vi "Telemetria+Datalogger.vi"() -> ()   [LabVIEW 2018]
uses:
  <vilib>/Utility/file.llb/Write Delimited Spreadsheet (string).vi
  <vilib>/Instr/_visa.llb/VISA Configure Serial Port (Instr).vi
  <vilib>/Utility/file.llb/Write Delimited Spreadsheet (I64).vi
  <vilib>/MakerHub/LINX/LMH-LINX.lvlib
panel:
  out "ITA":dbl
  out "AFR":dbl
  out "ECUS":dbl
  in  "stop":bool
  in  "VISA resource name":refnum<visa-resource-name>
  out "Loop Rate (Hz)":u32
  in  "Tab Control":T1(tab)
  out "BATT":dbl(knob) scale=0.0..14.0
  out "RPM":dbl(knob) scale=0.0..10000.0
  out "VSS1":dbl(knob) scale=0.0..200.0
  out "BATC":dbl(knob) scale=0.0..10.0
  out "VO2":dbl(knob) scale=0.0..10.0
  out "FP1":dbl(knob) scale=0.0..10.0
  out "BARO":dbl(knob) scale=0.0..100.0
  out "MAP":dbl(knob) scale=0.0..10.0
  out "CLT":dbl(slide) scale=0.0..10.0
  out "MAT":dbl(slide) scale=0.0..10.0
  out "AFC":dbl(slide) scale=0.0..10.0
  out "ADC":dbl(slide) scale=0.0..100.0
  out "WC":dbl(slide) scale=0.0..100.0
  out "VE1":dbl(slide) scale=0.0..10.0
  out "VE2":dbl(slide) scale=0.0..10.0
  out "LOAD":dbl(slide) scale=0.0..100.0
  out "KNOCK":i32(graph)
  out "TPS":i32(graph)
  out "KNOCK":string
  out "BARO":string
  in  "offset BARO":i32
  out "MAP":string
  out "RPM":string
  in  "length RPM":i32
  in  "offset RPM":i32
  out "CLT":string
  out "TPS":string
  in  "length TPS":i32
  in  "offset TPS":i32
  out "BATT":string
  in  "length BATT":i32
  in  "offset BATT":i32
  in  "length KNOCK":i32
  in  "offset KNOCK":i32
  out "MAT":string
  in  "length MAT":i32
  in  "offset MAT":i32
  out "VSS1":string
  in  "length VSS1":i32
  in  "offset VSS1":i32
  in  "length MAP":i32
  in  "offset MAP":i32
  in  "length CLT":i32
  in  "offset  CLT":i32
  in  "length BARO":i32
  out "GEAR":string
  in  "length GEAR":i32
  in  "offset GEAR":i32
  out "ENGINE":string
  in  "length ENGINE":i32
  in  "offset ENGINE":i32
  out "read buffer":string
  out "FP1":string
  in  "length FP1":i32
  in  "offset FP1":i32
  out "ECUS":string
  in  "offset ECUS":i32
  in  "length ECUS":i32
  out "AFC":string
  in  "length AFC":i32
  in  "offset AFC":i32
  out "BATC":string
  in  "length BATC":i32
  in  "offset BATC":i32
  out "VO2":string
  in  "length VO2":i32
  in  "offset VO2":i32
  out "ADC":string
  in  "length ADC":i32
  in  "offset ADC":i32
  out "WC":string
  in  "length WC":i32
  in  "offset WC":i32
  out "VE1":string
  in  "length VE1":i32
  in  "offset VE1":i32
  out "VE2":string
  in  "length VE2":i32
  in  "offset VE2":i32
  out "LOAD":string
  in  "length LOAD":i32
  in  "offset LOAD":i32
  out "AFR":string
  in  "length AFR":i32
  in  "offset AFR":i32
  out "ITA":string
  in  "length ITA":i32
  in  "offset ITA":i32
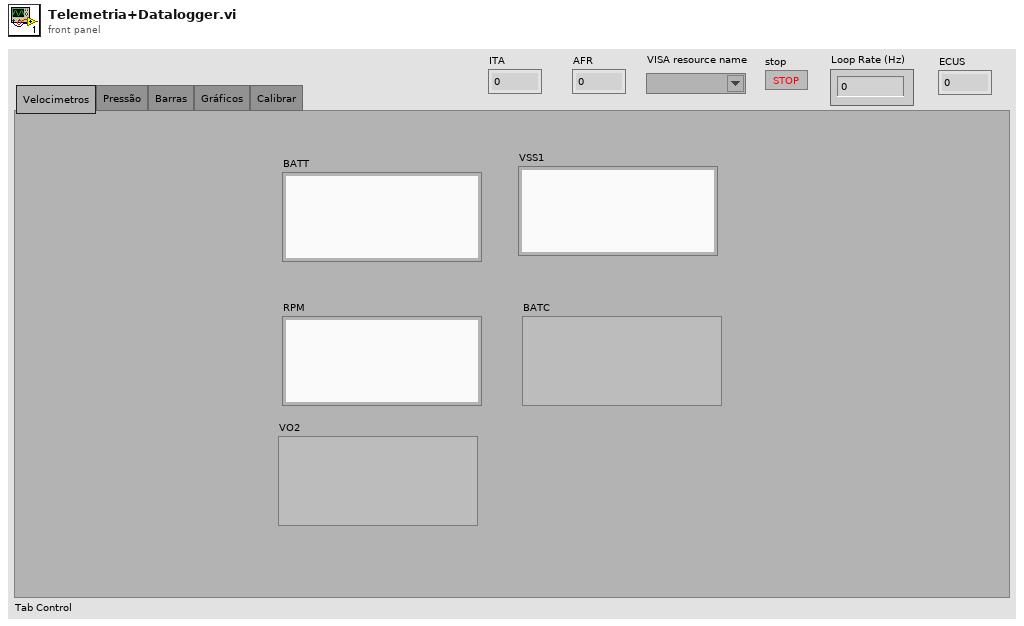
[diagram p1: front panel]
types:
  T1 = enum32{"Velocimetros", "Pressão", "Barras", "Gráficos", "Calibrar"}
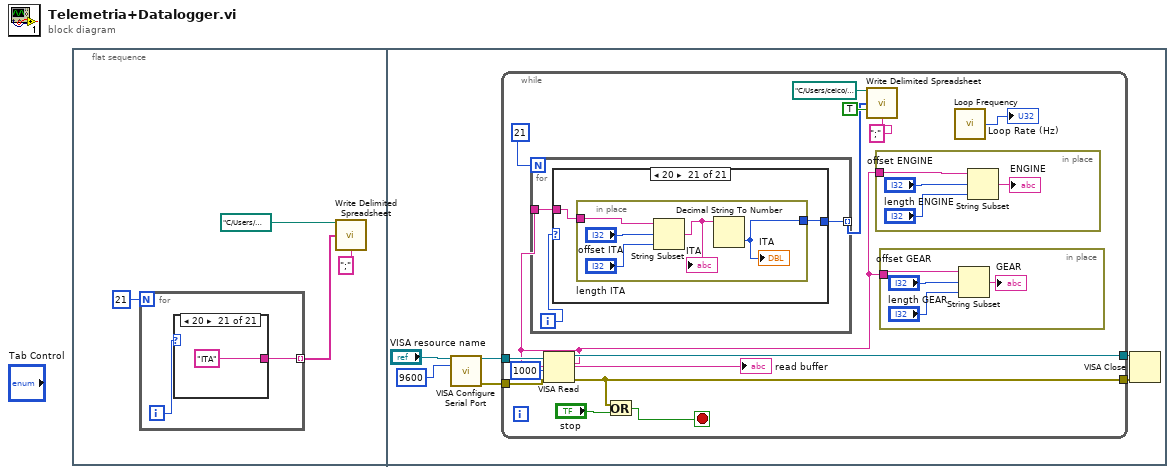
[diagram p0: block diagram]
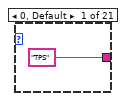
[diagram p2: hidden frame]
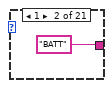
[diagram p3: hidden frame]
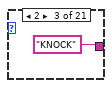
[diagram p4: hidden frame]
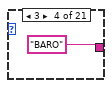
[diagram p5: hidden frame]
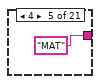
[diagram p6: hidden frame]
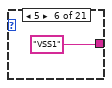
[diagram p7: hidden frame]
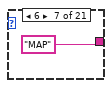
[diagram p8: hidden frame]
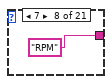
[diagram p9: hidden frame]
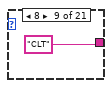
[diagram p10: hidden frame]
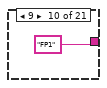
[diagram p11: hidden frame]
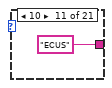
[diagram p12: hidden frame]
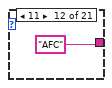
[diagram p13: hidden frame]
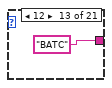
[diagram p14: hidden frame]
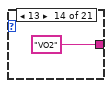
[diagram p15: hidden frame]
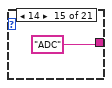
[diagram p16: hidden frame]
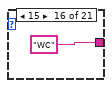
[diagram p17: hidden frame]
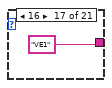
[diagram p18: hidden frame]
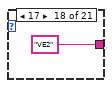
[diagram p19: hidden frame]
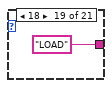
[diagram p20: hidden frame]
diagram:
  n1 = flat-sequence {
    frame #0 {
      n2 = for {
        N: 21 -> [_]
        tunnel: [w5] -> w2 mode=indexing
        i -> [w6]
        n3 = case shown="20" w6 {
          tunnel: ["TPS" "BATT" "KNOCK" "BARO" "MAT" "VSS1" "MAP" "RPM" "CLT" "FP1" "ECUS" "AFC" "BATC" "VO2" "ADC" "WC" "VE1" "VE2" "LOAD" "AFR" "ITA"] -> w5
          frame 0, Default {
          }
          frame 1 {
          }
          frame 2 {
          }
          frame 3 {
          }
          frame 4 {
          }
          frame 5 {
          }
          frame 6 {
          }
          frame 7 {
          }
          frame 8 {
          }
          frame 9 {
          }
          frame 10 {
          }
          frame 11 {
          }
          frame 12 {
          }
          frame 13 {
          }
          frame 14 {
          }
          frame 15 {
          }
          frame 16 {
          }
          frame 17 {
          }
          frame 18 {
          }
          frame 19 {
          }
          frame 20 {
          }
        }
      }
      n4 = call-poly <vilib>:"Write Delimited Spreadsheet.vi"("file path (dialog if empty)"=path "C:/Users/ceico/Documents/Scuderia/Telemetria/Teste Datalooger.csv", "1D data"=w2, "delimiter (\\t)"=";" ("delimiter (\\t)")) -> ()  [unwired: 11 in, 2 out]
    }
    frame #1 {
      n5 = call-poly "VISA Configure Serial Port"("VISA resource name"="VISA resource name", "baud rate (9600)"=u32 9600) -> ("VISA resource name out"=w30:refnum<visa-resource-name>, "error out"=w31:errorcluster)  [unwired: 12 in]
      n6 = while {
        tunnel: w30 -> [w45]
        tunnel: w31 -> [w44]
        tunnel: [w43] -> w32
        tunnel: [w42] -> w33
        stop <- w46 stop-if-true
        n7 = VISA Read(VISA resource name=w45, byte count=u32 1000, error in (no error)=w44) -> (VISA resource name out=w43:refnum<visa-resource-name>, read buffer=w34:string, error out=w42:errorcluster)  [unwired: 1 out]
        "read buffer" <- w34
        n8 = for {
          N: 21 -> [_]
          tunnel: w34 -> [w58]
          tunnel: [w56] -> w36 mode=indexing
          i -> [w57]
          n9 = case shown="20" w57 {
            tunnel: w58 -> [w60 w67 w74 w81 w87 w95 w102 w109 w116 w123 w130 w137 w144 w150 w158 w165 w172 w179 w186 w192 w200]
            tunnel: [w59 w66 w73 w80 w88 w94 w101 w108 w115 w122 w129 w136 w143 w151 w157 w164 w171 w178 w185 w193 w199] -> w56
            frame 0, Default {
              n10 = in-place {
                in-place-border: w60 -> [w62]
                in-place-border: [w61] -> w59
                n11 = String Subset(string=w62, offset (0)="offset TPS", length (rest)="length TPS") -> (substring=w65:string)
                "TPS" <- w65
                n12 = Decimal String To Number(string=w65) -> (number=w61:i32)  [unwired: 2 in, 1 out]
                "TPS" <- w61
              }
            }
            frame 1 {
              n13 = in-place {
                in-place-border: w67 -> [w69]
                in-place-border: [w68] -> w66
                n14 = String Subset(string=w69, offset (0)="offset BATT", length (rest)="length BATT") -> (substring=w72:string)
                "BATT" <- w72
                n15 = Decimal String To Number(string=w72) -> (number=w68:i32)  [unwired: 2 in, 1 out]
                "BATT" <- w68
              }
            }
            frame 2 {
              n16 = in-place {
                in-place-border: w74 -> [w76]
                in-place-border: [w75] -> w73
                n17 = String Subset(string=w76, offset (0)="offset KNOCK", length (rest)="length KNOCK") -> (substring=w79:string)
                "KNOCK" <- w79
                n18 = Decimal String To Number(string=w79) -> (number=w75:i32)  [unwired: 2 in, 1 out]
                "KNOCK" <- w75
              }
            }
            frame 3 {
              n19 = in-place {
                in-place-border: w81 -> [w83]
                in-place-border: [w82] -> w80
                n20 = String Subset(string=w83, offset (0)="offset BARO", length (rest)="length BARO") -> (substring=w86:string)
                "BARO" <- w86
                n21 = Decimal String To Number(string=w86) -> (number=w82:i32)  [unwired: 2 in, 1 out]
                "BARO" <- w82
              }
            }
            frame 4 {
              n22 = in-place {
                in-place-border: [w90] -> w88
                in-place-border: w87 -> [w89]
                n23 = String Subset(string=w89, offset (0)="offset MAT", length (rest)="length MAT") -> (substring=w93:string)
                "MAT" <- w93
                n24 = Decimal String To Number(string=w93) -> (number=w90:i32)  [unwired: 2 in, 1 out]
                "MAT" <- w90
              }
            }
            frame 5 {
              n25 = in-place {
                in-place-border: w95 -> [w97]
                in-place-border: [w96] -> w94
                n26 = String Subset(string=w97, offset (0)="offset VSS1", length (rest)="length VSS1") -> (substring=w100:string)
                "VSS1" <- w100
                n27 = Decimal String To Number(string=w100) -> (number=w96:i32)  [unwired: 2 in, 1 out]
                "VSS1" <- w96
              }
            }
            frame 6 {
              n28 = in-place {
                in-place-border: w102 -> [w104]
                in-place-border: [w103] -> w101
                n29 = String Subset(string=w104, offset (0)="offset MAP", length (rest)="length MAP") -> (substring=w107:string)
                "MAP" <- w107
                n30 = Decimal String To Number(string=w107) -> (number=w103:i32)  [unwired: 2 in, 1 out]
                "MAP" <- w103
              }
            }
            frame 7 {
              n31 = in-place {
                in-place-border: w109 -> [w111]
                in-place-border: [w110] -> w108
                n32 = String Subset(string=w111, offset (0)="offset RPM", length (rest)="length RPM") -> (substring=w114:string)
                "RPM" <- w114
                n33 = Decimal String To Number(string=w114) -> (number=w110:i32)  [unwired: 2 in, 1 out]
                "RPM" <- w110
              }
            }
            frame 8 {
              n34 = in-place {
                in-place-border: w116 -> [w118]
                in-place-border: [w117] -> w115
                n35 = String Subset(string=w118, offset (0)="offset  CLT", length (rest)="length CLT") -> (substring=w121:string)
                "CLT" <- w121
                n36 = Decimal String To Number(string=w121) -> (number=w117:i32)  [unwired: 2 in, 1 out]
                "CLT" <- w117
              }
            }
            frame 9 {
              n37 = in-place {
                in-place-border: w123 -> [w125]
                in-place-border: [w124] -> w122
                n38 = String Subset(string=w125, offset (0)="offset FP1", length (rest)="length FP1") -> (substring=w128:string)
                "FP1" <- w128
                n39 = Decimal String To Number(string=w128) -> (number=w124:i32)  [unwired: 2 in, 1 out]
                "FP1" <- w124
              }
            }
            frame 10 {
              n40 = in-place {
                in-place-border: w130 -> [w132]
                in-place-border: [w131] -> w129
                n41 = String Subset(string=w132, offset (0)="offset ECUS", length (rest)="length ECUS") -> (substring=w135:string)
                "ECUS" <- w135
                n42 = Decimal String To Number(string=w135) -> (number=w131:i32)  [unwired: 2 in, 1 out]
                "ECUS" <- w131
              }
            }
            frame 11 {
              n43 = in-place {
                in-place-border: w137 -> [w139]
                in-place-border: [w138] -> w136
                n44 = String Subset(string=w139, offset (0)="offset AFC", length (rest)="length AFC") -> (substring=w142:string)
                "AFC" <- w142
                n45 = Decimal String To Number(string=w142) -> (number=w138:i32)  [unwired: 2 in, 1 out]
                "AFC" <- w138
              }
            }
            frame 12 {
              n46 = in-place {
                in-place-border: w144 -> [w146]
                in-place-border: [w145] -> w143
                n47 = String Subset(string=w146, offset (0)="offset BATC", length (rest)="length BATC") -> (substring=w149:string)
                "BATC" <- w149
                n48 = Decimal String To Number(string=w149) -> (number=w145:i32)  [unwired: 2 in, 1 out]
                "BATC" <- w145
              }
            }
            frame 13 {
              n49 = in-place {
                in-place-border: w150 -> [w153]
                in-place-border: [w152] -> w151
                n50 = String Subset(string=w153, offset (0)="offset VO2", length (rest)="length VO2") -> (substring=w156:string)
                "VO2" <- w156
                n51 = Decimal String To Number(string=w156) -> (number=w152:i32)  [unwired: 2 in, 1 out]
                "VO2" <- w152
              }
            }
            frame 14 {
              n52 = in-place {
                in-place-border: w158 -> [w160]
                in-place-border: [w159] -> w157
                n53 = String Subset(string=w160, offset (0)="offset ADC", length (rest)="length ADC") -> (substring=w163:string)
                "ADC" <- w163
                n54 = Decimal String To Number(string=w163) -> (number=w159:i32)  [unwired: 2 in, 1 out]
                "ADC" <- w159
              }
            }
            frame 15 {
              n55 = in-place {
                in-place-border: w165 -> [w167]
                in-place-border: [w166] -> w164
                n56 = String Subset(string=w167, offset (0)="offset WC", length (rest)="length WC") -> (substring=w170:string)
                "WC" <- w170
                n57 = Decimal String To Number(string=w170) -> (number=w166:i32)  [unwired: 2 in, 1 out]
                "WC" <- w166
              }
            }
            frame 16 {
              n58 = in-place {
                in-place-border: w172 -> [w174]
                in-place-border: [w173] -> w171
                n59 = String Subset(string=w174, offset (0)="offset VE1", length (rest)="length VE1") -> (substring=w177:string)
                "VE1" <- w177
                n60 = Decimal String To Number(string=w177) -> (number=w173:i32)  [unwired: 2 in, 1 out]
                "VE1" <- w173
              }
            }
            frame 17 {
              n61 = in-place {
                in-place-border: w179 -> [w181]
                in-place-border: [w180] -> w178
                n62 = String Subset(string=w181, offset (0)="offset VE2", length (rest)="length VE2") -> (substring=w184:string)
                "VE2" <- w184
                n63 = Decimal String To Number(string=w184) -> (number=w180:i32)  [unwired: 2 in, 1 out]
                "VE2" <- w180
              }
            }
            frame 18 {
              n64 = in-place {
                in-place-border: w186 -> [w188]
                in-place-border: [w187] -> w185
                n65 = String Subset(string=w188, offset (0)="offset LOAD", length (rest)="length LOAD") -> (substring=w191:string)
                "LOAD" <- w191
                n66 = Decimal String To Number(string=w191) -> (number=w187:i32)  [unwired: 2 in, 1 out]
                "LOAD" <- w187
              }
            }
            frame 19 {
              n67 = in-place {
                in-place-border: w192 -> [w195]
                in-place-border: [w194] -> w193
                n68 = String Subset(string=w195, offset (0)="offset AFR", length (rest)="length AFR") -> (substring=w198:string)
                "AFR" <- w198
                n69 = Decimal String To Number(string=w198) -> (number=w194:i32)  [unwired: 2 in, 1 out]
                "AFR" <- w194
              }
            }
            frame 20 {
              n70 = in-place {
                in-place-border: w200 -> [w202]
                in-place-border: [w201] -> w199
                n71 = String Subset(string=w202, offset (0)="offset ITA", length (rest)="length ITA") -> (substring=w205:string)
                "ITA" <- w205
                n72 = Decimal String To Number(string=w205) -> (number=w201:i32)  [unwired: 2 in, 1 out]
                "ITA" <- w201
              }
            }
          }
        }
        n73 = Or(x=w42, y="stop") -> (x .or. y?=w46:bool)
        n74 = call-poly <vilib>:"Write Delimited Spreadsheet.vi"("file path (dialog if empty)"=path "C:/Users/ceico/Documents/Scuderia/Telemetria/Teste Datalooger.csv", "1D data"=w36, "append to file? (new file:F)"=TRUE, "delimiter (\\t)"=";" ("delimiter (\\t)")) -> ()  [unwired: 10 in, 2 out]
        n75 = in-place {
          in-place-border: w34 -> [w52]
          n76 = String Subset(string=w52, offset (0)="offset ENGINE", length (rest)="length ENGINE") -> (substring=→"ENGINE":string)
        }
        n77 = in-place {
          in-place-border: w34 -> [w48]
          n78 = String Subset(string=w48, offset (0)="offset GEAR", length (rest)="length GEAR") -> (substring=→"GEAR":string)
        }
        n79 = call <vilib>:"Loop Frequency.vi"() -> ("Loop Rate (Hz)"=→"Loop Rate (Hz)":u32)
      }
      n80 = VISA Close(VISA resource name=w32, error in (no error)=w33) -> ()  [unwired: 1 out]
    }
  }
